vi "Setup camera (SubVI).vi"(4 "M duty cycle [P]":dbl=533.0 format="%#_13g", 5 "S duty cycle [B]   in":dbl=990.0 format="%#_13g", 6 "M duty cycle [B]  in":dbl=533.0 format="%#_13g", 7 "S duty cycle [F]":dbl=620.0 format="%#_13g", 9 "M duty cycle [F]":dbl=506.0 format="%#_13g", 10 "Camera state":enum16{"Fwd", "Pattern", "Ball"}(ring), 11 "S duty cycle [P]":dbl=990.0 format="%#_13g") -> (2 "M duty cycle [B]  out":dbl, 3 "S duty cycle [B]   out":dbl)   [LabVIEW 2017]
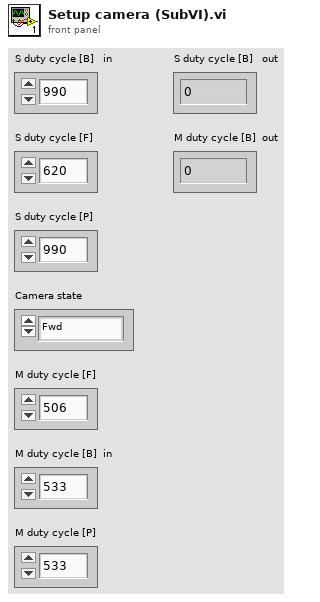
[diagram p1: front panel]
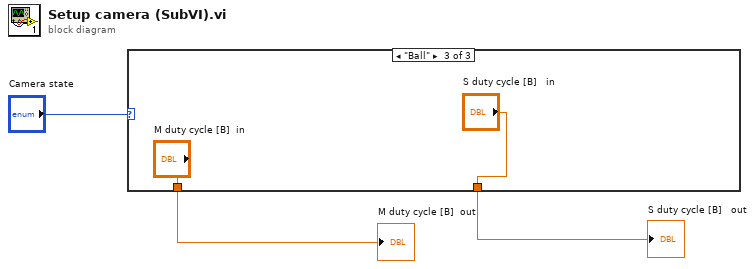
[diagram p0: block diagram]
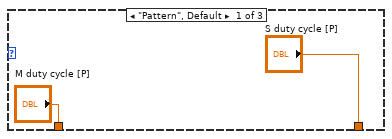
[diagram p2: hidden frame]
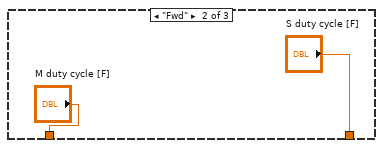
[diagram p3: hidden frame]
diagram:
  n1 = case shown="\"Ball\"" "Camera state" {
    tunnel: ["S duty cycle [P]" "S duty cycle [F]" "S duty cycle [B]   in"] -> w3
    tunnel: ["M duty cycle [P]" "M duty cycle [F]" "M duty cycle [B]  in"] -> w2
    frame "Pattern", Default {
    }
    frame "Fwd" {
    }
    frame "Ball" {
    }
  }
  "S duty cycle [B]   out" <- w3
  "M duty cycle [B]  out" <- w2
